vi "Role Decisors Selector.vi"(0 "Receptor passe":enum16{"Auto", "2nd Striker", "Striker"}(ring), 4 "IA State Output":T2 {"enemy_robots"."Agentes Disponíveis" format="%#_13g"; "our_robots"."Agentes Disponíveis" format="%#_13g"}, 5 "InfoMissao":T13 {"Agentes Disponíveis" format="%#_13g"}, 6 "Pinned":T14={"Attc"="Auto", "Strk"="Auto", "Def"=[], "Strk 2"="Auto"}, 7 "Qtd Min p/\n2nd Stk":i32=5, 8 "Modo Teste ?":bool, 9 "Qtd Min p/ Stk":i32=2, 10 "Role Decisor":T17(ring), 11 "channel":T16) -> (1 "channel info":T1, 2 "Output IA":T2 {"enemy_robots"."Agentes Disponíveis" format="%#_13g"; "our_robots"."Agentes Disponíveis" format="%#_13g"}, 3 "channel":T16)   [LabVIEW 2018]
uses:
  <extravilib>/ChannelInstances/Lossy Stream-t'AI Input.ctl'/)Channel.ctl
  Core/AI Input.ctl
  Core/AI Robot.ctl
  Intel/Functions Enum.ctl
  Intel/AttackerStates.ctl
  Path Planning/RRT/PathDests.ctl
  Path Planning/RRT/PathDest.ctl
  Core/AI Ball.ctl
  Core/Field Size.ctl
  Core/AI Judge.ctl
  Intel/Command Enum.ctl
  Util/Events/Events.ctl
  Select Personalitys.ctl
  Util/Select Auto None or Robot.ctl
  InfoMissao.ctl
  <extravilib>/ChannelInstances/Lossy Stream-t'InfoMissao.ctl'/)Channel.ctl
  <extravilib>/ChannelInstances/Lossy Stream-t'AI Input.ctl'.lvlib
  <extravilib>/ChannelInstances/Lossy Stream-t'InfoMissao.ctl'.lvlib
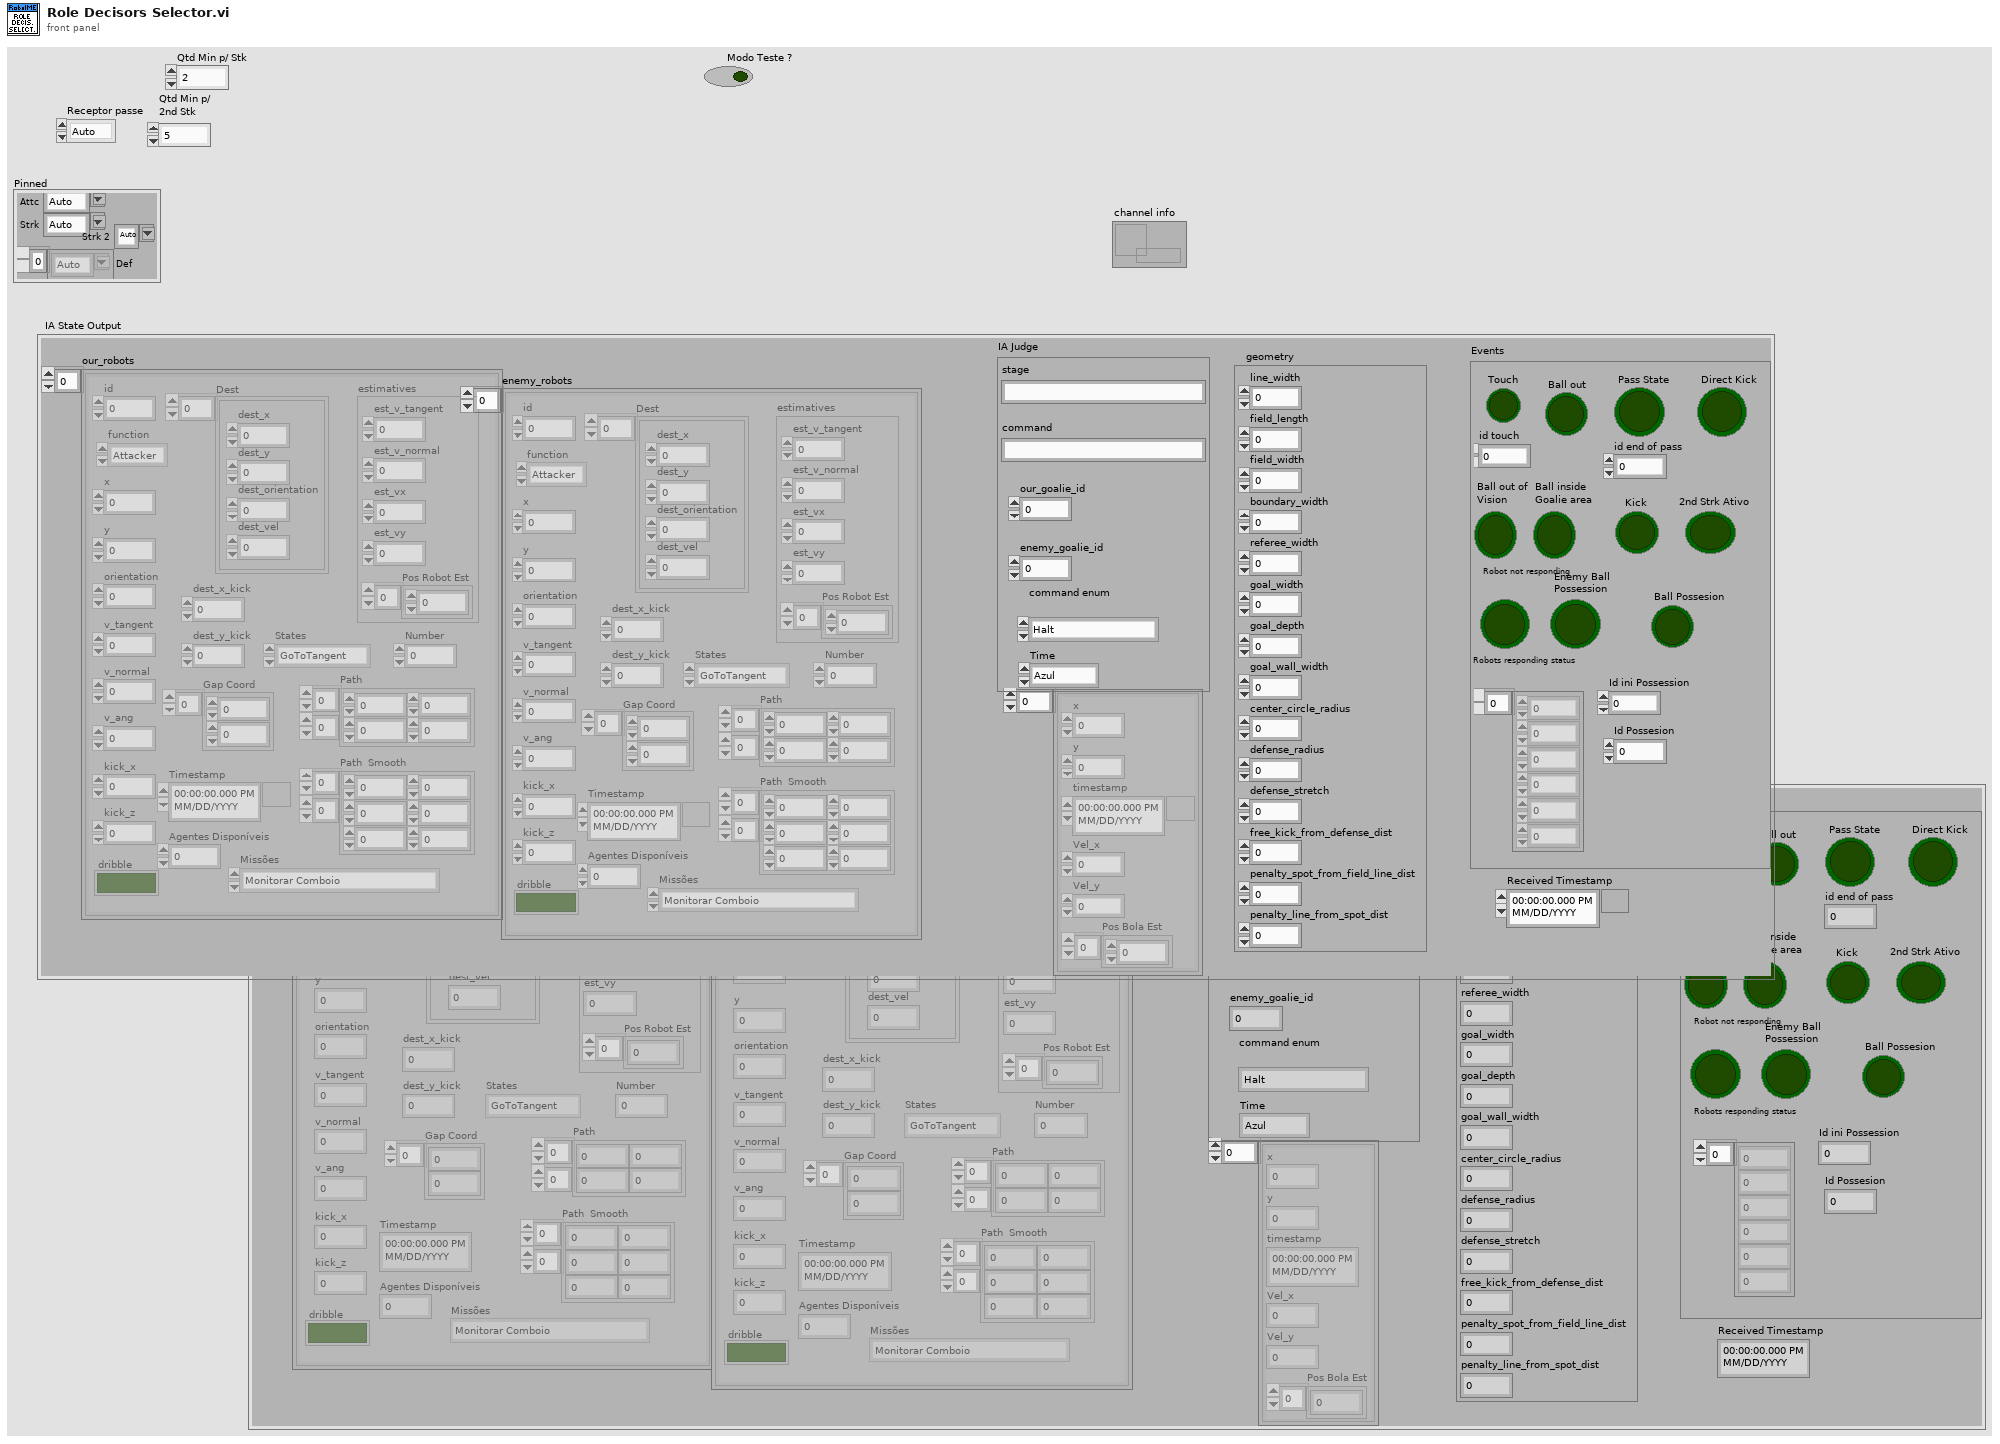
[diagram p1: front panel]
types:
  T1 = typedef "Lossy Stream-t'InfoMissao.ctl'.lvlib/)Channel.ctl" = refnum<queue>
  T2 = typedef "AI Input.ctl" = cluster{"our_robots":T3[], "enemy_robots":T3[], "balls":T8[], "geometry":T9, "IA Judge":T10, "Received Timestamp":timestamp, "Events":T12}
  T3 = typedef "AI Robot.ctl" = cluster{"id":u32, "function":T4, "x":dbl, "y":dbl, "orientation":dbl, "v_tangent":dbl, "v_normal":dbl, "v_ang":dbl, "kick_x":dbl, "kick_z":dbl, "dribble":bool, "Timestamp":timestamp, "estimatives":cluster{"est_v_tangent":dbl, "est_v_normal":dbl, "est_vx":dbl, "est_vy":dbl, "Pos Robot Est":dbl[]}, "dest_x_kick":dbl, "dest_y_kick":dbl, "Gap Coord":dbl[], "States":T5, "Path ":dbl[][], "Path  Smooth":dbl[][], "Dest":T6, "Missões ":enum16{"Monitorar Comboio", "Realizar Segurança de Retaguarda", "Vigiar Área", "Reconhecimento de Área"}, "Agentes Disponíveis":dbl, "Number":dbl}
  T4 = typedef "Functions Enum.ctl" = enum16{"None", "Vigia", "2nd Striker", "Attacker", "Goalie", "Defender", "Striker", "Goto 0", "Dummy", "Kicker", "ZigZag 0", "ZigZag 1", "ZigZag 2", "ZigZag 3", "ZigZag 4", "ZigZag 5", "ZigZag 6", "ZigZag 7", "ZigZag 8", ""}
  T5 = typedef "AttackerStates.ctl" = enum16{"Pass", "GoToTangent", "BallGetting", "GoToKick", ""}
  T6 = typedef "PathDests.ctl" = T7[]
  T7 = typedef "PathDest.ctl" = cluster{"dest_x":dbl, "dest_y":dbl, "dest_orientation":dbl, "dest_vel":dbl}
  T8 = typedef "AI Ball.ctl" = cluster{"x":dbl, "y":dbl, "timestamp":timestamp, "Vel_x":dbl, "Vel_y":dbl, "Pos Bola Est":dbl[]}
  T9 = typedef "Field Size.ctl" = cluster{"line_width":u32, "field_length":u32, "field_width":u32, "boundary_width":u32, "referee_width":u32, "goal_width":u32, "goal_depth":u32, "goal_wall_width":u32, "center_circle_radius":u32, "defense_radius":u32, "defense_stretch":u32, "free_kick_from_defense_dist":u32, "penalty_spot_from_field_line_dist":u32, "penalty_line_from_spot_dist":u32}
  T10 = typedef "AI Judge.ctl" = cluster{"stage":string, "command":string, "our_goalie_id":dbl, "enemy_goalie_id":dbl, "command enum":T11, "Time":enum16{"Azul", "Amarelo"}}
  T11 = typedef "Command Enum.ctl" = enum16{"Halt", "Stop", "Force Start", "PKA Normal Start", "Prepare Kickoff Ally", "PKE Normal Start", "Prepare Kickoff Enemy", "Prepare Penalty Ally", "PPA Normal Start", "Prepare Penalty Enemy", "PPE Normal Start", "Direct Free Enemy", "Direct Free Ally", "Indirect Free Enemy", "Indirect Free Ally", "Timeout Enemy", "Timeout Ally", "Goal Enemy", "Goal Ally", "Ball Placement Enemy", "Ball Placement Ally", "Normal Half Time", "Extra Time Break", "Extra Half Time", "None", "Post Game"}
  T12 = typedef "Events.ctl" = cluster{"Touch":bool, "Ball out":bool, "id touch":dbl, "Ball out of \nVision":bool, "Ball inside \nGoalie area":bool, "Robot not responding":bool, "Robots responding status":dbl[], "Enemy Ball \nPossession":bool, "Pass State":bool, "id end of pass":dbl, "Kick":bool, "Id ini Possession":dbl, "Ball Possesion":bool, "Id Possesion":dbl, "Direct Kick":bool, "2nd Strk Ativo":bool}
  T13 = typedef "InfoMissao.ctl" = cluster{"Troca ":bool, "Missões ":enum16{"Monitorar Comboio", "Realizar Segurança de Retaguarda", "Vigiar Área", "Reconhecimento de Área"}, "Agentes Disponíveis":dbl, "id troca ":dbl, "id subs":dbl}
  T14 = typedef "Select Personalitys.ctl" = cluster{"Attc":T15, "Strk":T15, "Def":T15[], "Strk 2":T15}
  T15 = typedef "Select Auto None or Robot.ctl" = string
  T16 = typedef "Lossy Stream-t'AI Input.ctl'.lvlib/)Channel.ctl" = refnum<queue>
  T17 = enum16{"Simple Role Decisor", "PFC Role Decisor", "No Role Decisor"}
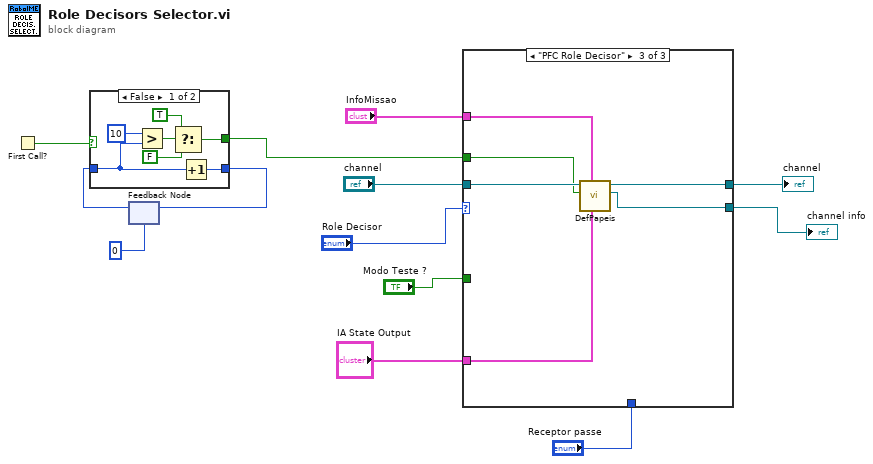
[diagram p0: block diagram]
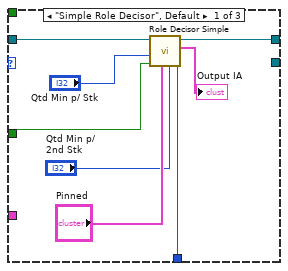
[diagram p3: hidden frame]
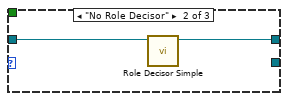
[diagram p4: hidden frame]
diagram:
  n1 = First Call?() -> (First Call?: T/F=w5:bool)
  n2 = feedback #1(0) -> (w4:i32)
  n3 = case shown="False" w5 {
    selector: w5 -> [_ w21]
    tunnel: w4 -> [w14 w22]
    tunnel: [w15 w22] -> w6
    tunnel: [w20 w21] -> w2
    frame False {
      n4 = Greater?(x=10, y=w14) -> (0:w19:bool)
      n5 = Select(t=TRUE, s=w19, f=FALSE) -> (s? t:f=w20:bool)
      n6 = Increment(x=w14) -> (x+1=w15:i32)
    }
    frame True {
    }
  }
  n7 = feedback-in #1(w6) -> ()
  n8 = case shown="\"PFC Role Decisor\"" "Role Decisor" {
    tunnel: "channel" -> [w30 w32 w38]
    tunnel: [w29 w31 w37] -> w12
    tunnel: "Modo Teste ?" -> [w26 _ _]
    tunnel: "Receptor passe" -> [w24 _ _]
    tunnel: "InfoMissao" -> [_ _ w36]
    tunnel: "IA State Output" -> [_ _ w35]
    tunnel: w2 -> [_ _ w34]
    tunnel: [_ _ w33] -> w1
    frame "Simple Role Decisor", Default {
      n9 = call "Role Decisor Simple.vi"("Receptor passe"=w24, "Qtd Min p/\n2nd Stk"="Qtd Min p/\n2nd Stk", "Pinned"="Pinned", "Modo Teste ?"=w26, "Qtd Min p/ Stk"="Qtd Min p/ Stk", "channel"=w30) -> ("Output IA"=→"Output IA":T2, "channel 2"=w29:T16)  [unwired: 4 in]
    }
    frame "No Role Decisor" {
      n10 = call "Role Decisor Simple.vi"("channel"=w32) -> ("channel 2"=w31:T16)  [unwired: 9 in, 1 out]
    }
    frame "PFC Role Decisor" {
      n11 = call "DefPapeis.vi"("IA State Output"=w35, "InfoMissao"=w36, "Boolean"=w34, "channel"=w38) -> ("channel info"=w33:T1, "channel 2"=w37:T16)  [unwired: 6 in]
    }
  }
  "channel" <- w12
  "channel info" <- w1
